vi "JSONtext API example.vi"() -> ()   [LabVIEW 2017]
doc: "Basic JSONtext example, showing multiple ways of using the API, including using JSON Path notation."
uses:
  JSON Value Type.ctl
  43bbaf7c-91b5-4e1a-837b-f8a4a49da893.vi
  ad9ae1fd-b9d5-4f13-a92f-47e516535324.vi
  5d88fb63-8c91-44b3-9a4f-d3581fd2733f.vi
  254eee29-e9a7-45f4-95fc-98b1af8f77a9.vi
  bed1c04e-f31b-4ea7-8c25-aae623e50321.vi
  efc312b2-f90b-47d6-8d2c-b412d5718184.vi
  833036be-c5ea-43e7-9d68-87ff15d910d2.vi
  247491b2-9e92-4ce0-aad1-0a934daafb37.vi
  365b7ad2-582b-481d-b7ea-7f90626a90ef.vi
  cd823ea4-ae16-4df6-9e87-f90ee35a06a1.vi
  b29da72e-adf8-46d7-b39b-1f679b2d23b5.vi
  a6b62a41-ffb4-49a5-9615-10447676f114.vi
  String Subset.vi
  Find Multiple Items.vi
  support/Quote and Escape JSON string.vi
  support/Strip Quotes and Unescape.vi
  support/quote and escape json string 2.vi
  Variant to JSON Text.vi
  Set Multiple Object Items.vi
  Parsing/Parse Full Path or Item Name.vi
  Offset/Find Item Locations by Path.vi
  support/Unescape JSON string.vi
  JSON text to Variant.vi
  Offset/Find Object Item Locations by Names.vi
  JSONtext.lvlib
panel:
  out "relayed_by":string
  out "size":i32
  out "JSON Value Type":T1
  in  "Pretty Print Levels":i32=6
  out "<JSON> 2":string[](array[string]) caption="Found in x object"
  out "All (incl. Added Array)":T2
  out "out":T3(array[cluster])
  out "x.inputs.prev_out.addr":string[](array[string])
  out "x.vin_sz":i32[](array[numeric])
  in  "Added Array Size":i32=10
  in  "Test Cluster":T4={"op"="utx", "x"={"lock_time"=0, "ver"=1, "size"=192, "inputs"=[{"sequence"=4294967295, "prev_out"={"spent"=TRUE, "tx_index"=99005468, "type"=0, "addr"="1BwGf3z7n2fHk6NoVJNkV32qwyAYsMhkWf", "value"=65574000, "n"=0, "script"="76a91477f4c9ee75e449a74c21a4decfb50519cbc245b388ac"}, "script"="483045022100e4ff962c292705f051c2c2fc519fa775a4d8955bce1a3e29884b2785277999ed02200b537ebd22a9f25fbbbcc9113c69c1389400703ef2017d80959ef0f1d685756c012102618e08e0c8fd4c5fe539184a30fe35a2f5fccf7ad62054cad29360d871f8187d"}, {"sequence"=22222222, "prev_out"={"spent"=TRUE, "tx_index"=99005469, "type"=1, "addr"="Blah Blah Blah", "value"=222222, "n"=0, "script"="76a91477f4c9ee75e449a74c21a4decfb50519cbc245b388ac"}, "script"="483045022100e4ff962c292705f051c2c2fc519fa775a4d8955bce1a3e29884b2785277999ed02200b537ebd22a9f25fbbbcc9113c69c1389400703ef2017d80959ef0f1d685756c012102618e08e0c8fd4c5fe539184a30fe35a2f5fccf7ad62054cad29360d871f8187d"}], "time"=1440086763, "tx_index"=99006637, "vin_sz"=1, "hash"="0857b9de1884eec314ecf67c040a2657b8e083e1f95e31d0b5ba3d328841fc7f", "vout_sz"=1, "relayed_by"="127.0.0.1", "out"=[{"spent"=FALSE, "tx_index"=99006637, "type"=0, "addr"="1A828tTnkVFJfSvLCqF42ohZ51ksS3jJgX", "value"=65564000, "n"=0, "script"="76a914640cfdf7b79d94d1c980133e3587bd6053f091f388ac"}, {"spent"=TRUE, "tx_index"=123, "type"=0, "addr"="1A828tTnkVFJfSvLCqF42ohZ51ksS3jJgX", "value"=13234312, "n"=1, "script"="76a914640cfdf7b79d94d1c980133e3587bd6053f091f388ac"}]}}
  out "<JSON>":string
  # "Run this VI, then see block diagram:"
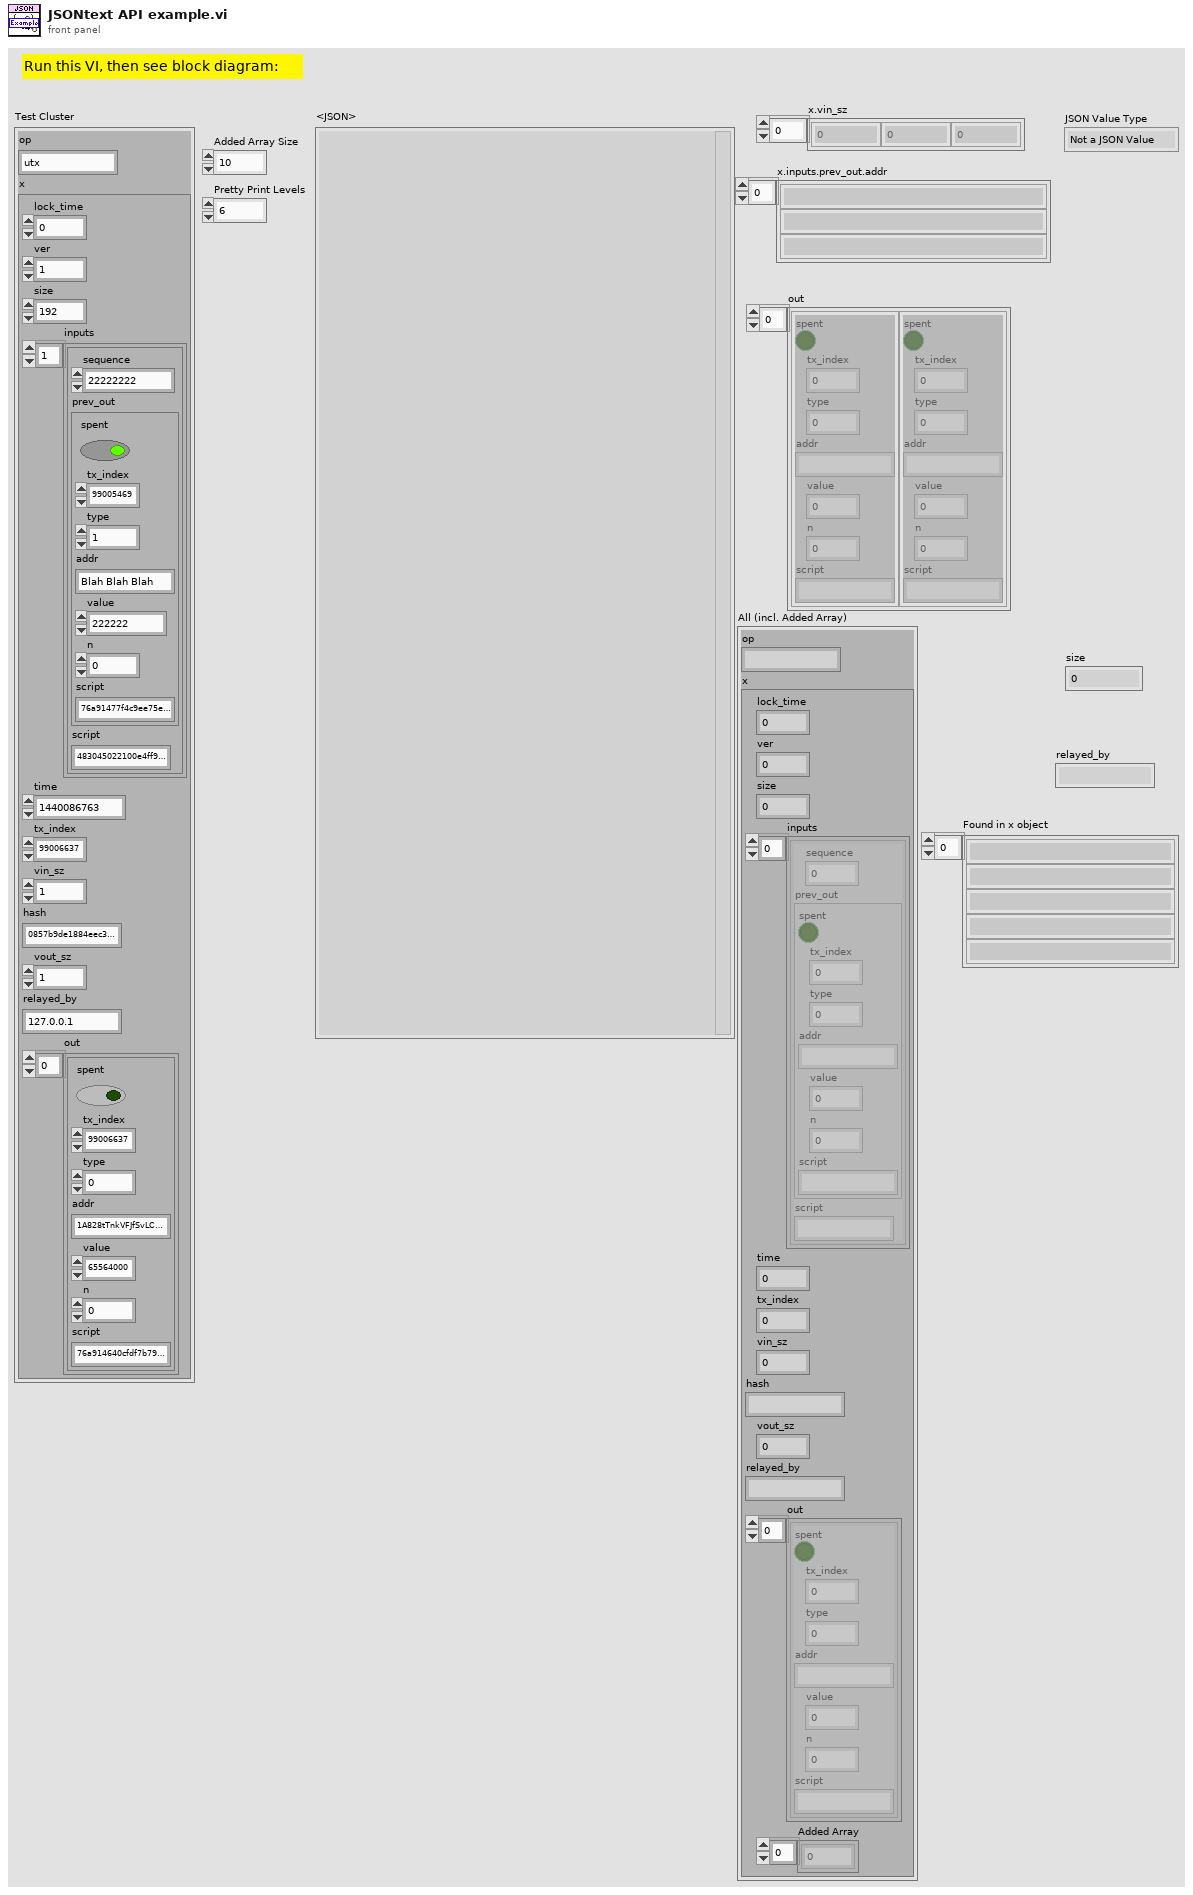
[diagram p1: front panel]
types:
  T1 = typedef "JSONtext.lvlib/JSON Value Type.ctl" = enum16{"Not a JSON Value", "JSON Object", "JSON Array", "String", "Number", "true", "false", "null"}
  T2 = cluster{"op":string, "x":cluster{"lock_time":i32, "ver":i32, "size":i32, "inputs":cluster{"sequence":i64, "prev_out":cluster{"spent":bool, "tx_index":i32, "type":i32, "addr":string, "value":i32, "n":i32, "script":string}, "script":string}[], "time":i32, "tx_index":i32, "vin_sz":i32, "hash":string, "vout_sz":i32, "relayed_by":string, "out":cluster{"spent":bool, "tx_index":i32, "type":i32, "addr":string, "value":i32, "n":i32, "script":string}[], "Added Array":dbl[]}}
  T3 = cluster{"spent":bool, "tx_index":i32, "type":i32, "addr":string, "value":i32, "n":i32, "script":string}[]
  T4 = cluster{"op":string, "x":cluster{"lock_time":i32, "ver":i32, "size":i32, "inputs":cluster{"sequence":i64, "prev_out":cluster{"spent":bool, "tx_index":i32, "type":i32, "addr":string, "value":i32, "n":i32, "script":string}, "script":string}[], "time":i32, "tx_index":i32, "vin_sz":i32, "hash":string, "vout_sz":i32, "relayed_by":string, "out":cluster{"spent":bool, "tx_index":i32, "type":i32, "addr":string, "value":i32, "n":i32, "script":string}[]}}
  T5 = cluster{"size":i32, "relayed_by":string, "out":cluster{"spent":bool, "tx_index":i32, "type":i32, "addr":string, "value":i32, "n":i32, "script":string}[]}
  T6 = cluster{"Merged String":string, "Merged Number":i32, "seconds since 1Jan1904":timestamp, "date string":string, "time string":string}
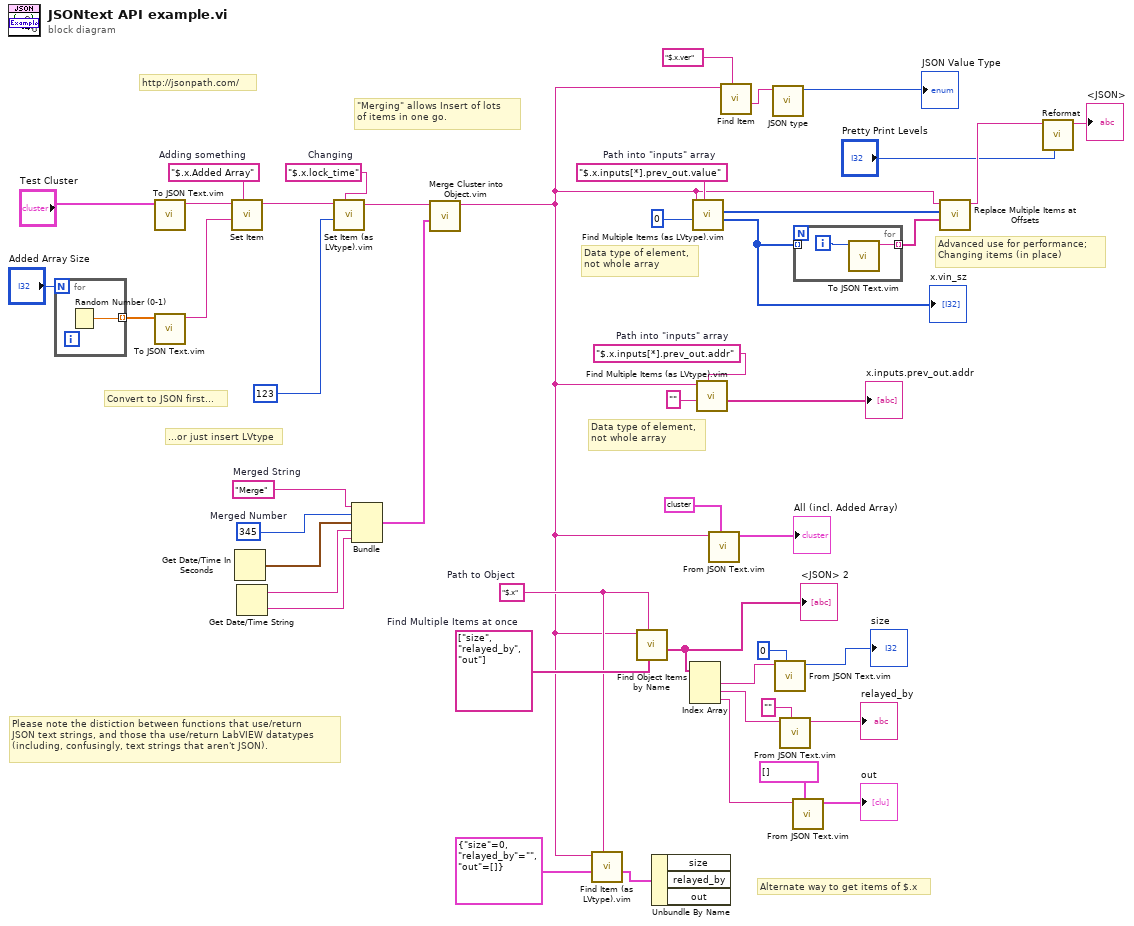
[diagram p0: block diagram]
diagram:
  w19 = 345  # Merged Number
  w20 = "Merge"  # Merged String
  w38 = string[] ["size", "relayed_by", "out"]  # Find Multiple Items at once
  w23 = "$.x"  # Path to Object
  w25 = "$.x.inputs[*].prev_out.addr"  # Path into "inputs" array
  w39 = "$.x.inputs[*].prev_out.value"  # Path into "inputs" array
  w41 = "$.x.lock_time"  # Changing
  w45 = "$.x.Added Array"  # Adding something
  # "Please note the distiction between functions that use/return\nJSON text strings, and those tha use/return LabVIEW datatypes\n(including, confusingly, text strings that aren't JSON)."
  # "Data type of element,\nnot whole array"
  # "\"Merging\" allows Insert of lots \nof items in one go."
  # "Data type of element,\nnot whole array"
  # "Alternate way to get items of $.x"
  # "...or just insert LVtype"
  # "Convert to JSON first..."
  # "Advanced use for performance;\nChanging items (in place)"
  # "http://jsonpath.com/"
  n1 = for {
    N: "Added Array Size" -> [_]
    tunnel: [w48] -> w43 mode=indexing
    n2 = Random Number (0-1)() -> (number: 0 to 1=w48:dbl)
  }
  n3 = call "To JSON Text.vim"("Anything"="Test Cluster") -> ("<JSON>"=w46:string)  [unwired: 9 in, 1 out]
  n4 = call "To JSON Text.vim"("Anything"=w43) -> ("<JSON>"=w37:string)  [unwired: 9 in, 1 out]
  n5 = call "Set Item.vi"("$Path or Item Name"=w45, "JSON to Insert"=w37, "JSON"=w46) -> ("<JSON>"=w42:string)  [unwired: 5 in, 2 out]
  n6 = Get Date/Time In Seconds() -> (seconds since 1Jan1904=w17:timestamp)
  n7 = Get Date/Time String() -> (date string=w16:string, time string=w15:string)  [unwired: 3 in]
  n8 = call "Set Item (as LVtype).vim"("Object (or Item) Path"=w41, "Anything"=123, "JSON"=w42) -> ("<JSON>"=w21:string)  [unwired: 5 in, 2 out]
  n9 = Bundle("Merged String"=w20, "Merged Number"=w19, "seconds since 1Jan1904"=w17, "date string"=w16, "time string"=w15) -> (w18:T6)  [unwired: 1 in]
  n10 = call "Merge Cluster into Object.vim"("Any Cluster"=w18, "JSON"=w21) -> ("<JSON>"=w3:string)  [unwired: 7 in, 1 out]
  n11 = call "Find Item (as LVtype).vim"("$Path or Item Name"=w23, "Data Type and Default Value"=T5 {"size"=0, "relayed_by"="", "out"=[]}, "JSON"=w3) -> ("Data"=w14:T5)  [unwired: 5 in, 3 out]
  n12 = call "Find Object Items by Name.vi"("Item Names"=w38, "$Path or Item Name"=w23, "JSON"=w3) -> ("<JSON>"=w31:string[])  [unwired: 6 in, 2 out]
  "<JSON> 2" <- w31
  n13 = Unbundle By Name(w14) -> ()  [unwired: 3 out]
  n14 = Index Array(array=w31) -> (element #1=w28:string, element #2=w6:string, element #3=w5:string)  [unwired: 3 in]
  n15 = call "Find Multiple Items (as LVtype).vim"("$Path or Item Name"=w39, "Data Type and Default Value"=0 ("Number"), "JSON"=w3) -> ("Array of Data"=w9:i32[], "Item Offsets"=w36:i32[])  [unwired: 5 in, 2 out]
  "x.vin_sz" <- w9
  n16 = call "Find Multiple Items (as LVtype).vim"("$Path or Item Name"=w25, "Data Type and Default Value"="", "JSON"=w3) -> ("Array of Data"=→"x.inputs.prev_out.addr":string[])  [unwired: 5 in, 3 out]
  n17 = call "From JSON Text.vim"("Data Type and Default Value"=T2 {"op"="utx", "x"={"lock_time"=0, "ver"=1, "size"=192, "inputs"=[{"sequence"=4294967295, "prev_out"={"spent"=TRUE, "tx_index"=99005468, "type"=0, "addr"="1BwGf3z7n2fHk6NoVJNkV32qwyAYsMhkWf", "value"=65574000, "n"=0, "script"="76a91477f4c9ee75e449a74c21a4decfb50519cbc245b388ac"}, "script"="483045022100e4ff962c292705f051c2c2fc519fa775a4d8955bce1a3e29884b2785277999ed02200b537ebd22a9f25fbbbcc9113c69c1389400703ef2017d80959ef0f1d685756c012102618e08e0c8fd4c5fe539184a30fe35a2f5fccf7ad62054cad29360d871f8187d"}, {"sequence"=22222222, "prev_out"={"spent"=TRUE, "tx_index"=99005469, "type"=1, "addr"="Blah Blah Blah", "value"=222222, "n"=0, "script"="76a91477f4c9ee75e449a74c21a4decfb50519cbc245b388ac"}, "script"="483045022100e4ff962c292705f051c2c2fc519fa775a4d8955bce1a3e29884b2785277999ed02200b537ebd22a9f25fbbbcc9113c69c1389400703ef2017d80959ef0f1d685756c012102618e08e0c8fd4c5fe539184a30fe35a2f5fccf7ad62054cad29360d871f8187d"}], "time"=1440086763, "tx_index"=99006637, "vin_sz"=1, "hash"="0857b9de1884eec314ecf67c040a2657b8e083e1f95e31d0b5ba3d328841fc7f", "vout_sz"=1, "relayed_by"="127.0.0.1", "out"=[{"spent"=FALSE, "tx_index"=99006637, "type"=0, "addr"="1A828tTnkVFJfSvLCqF42ohZ51ksS3jJgX", "value"=65564000, "n"=0, "script"="76a914640cfdf7b79d94d1c980133e3587bd6053f091f388ac"}, {"spent"=TRUE, "tx_index"=123, "type"=0, "addr"="1A828tTnkVFJfSvLCqF42ohZ51ksS3jJgX", "value"=13234312, "n"=1, "script"="76a914640cfdf7b79d94d1c980133e3587bd6053f091f388ac"}], "Added Array"=[]}} ("Test Cluster"), "JSON"=w3) -> ("Data out"=→"All (incl. Added Array)":T2)  [unwired: 8 in, 1 out]
  n18 = call "Find Item.vi"("$Path or Item Name"="$.x.ver", "JSON"=w3) -> ("<JSON>"=w1:string)  [unwired: 6 in, 3 out]
  n19 = call "JSON type.vi"("JSON"=w1) -> ("JSON Value Type"=→"JSON Value Type":T1)  [unwired: 9 in, 1 out]
  n20 = call "From JSON Text.vim"("Data Type and Default Value"=0, "JSON"=w28) -> ("Data out"=→"size":i32)  [unwired: 8 in, 1 out]
  n21 = call "From JSON Text.vim"("Data Type and Default Value"="", "JSON"=w6) -> ("Data out"=→"relayed_by":string)  [unwired: 8 in, 1 out]
  n22 = call "From JSON Text.vim"("Data Type and Default Value"=T3 [], "JSON"=w5) -> ("Data out"=→"out":T3)  [unwired: 8 in, 1 out]
  n23 = for {
    tunnel: w9 -> [_] mode=indexing
    tunnel: [w50] -> w35 mode=indexing
    i -> [w49]
    n24 = call "To JSON Text.vim"("Anything"=w49) -> ("<JSON>"=w50:string)  [unwired: 9 in, 1 out]
  }
  n25 = call "Replace Multiple Items at Offsets.vi"("New JSON Items"=w35, "Offsets of Items to Replace"=w36, "JSON"=w3) -> ("<JSON>"=w34:string)  [unwired: 7 in, 1 out]
  n26 = call "Reformat.vi"("Pretty Print Levels"="Pretty Print Levels", "JSON"=w34) -> ("<JSON>First JSON Value\n\n<JSON>"=→"<JSON>":string)  [unwired: 6 in, 3 out]
